vi "Configure Session.vi"(8 "error in":errorcluster, 11 "Plugin in":refnum<class "Sift Stream.lvclass">) -> (0 "error out":errorcluster, 3 "Plugin out":refnum<class "Sift Stream.lvclass">)   [LabVIEW 2024, in "Sift Stream.lvlib" / "Sift Stream.lvclass"]
uses:
  Sift Stream.lvclass
  C:/Program Files/National Instruments/LabVIEW 2024/vi.lib/FlexLogger/SDK/PluginSDK.lvlibp/PEFClasses/SDK/Plugin/Plugin.lvclass
  <vilib>/FlexLogger/SDK/PluginSDK.lvlibp/PEFClasses/SDK/Processing Element/Timing Parameters.ctl
  <vilib>/FlexLogger/SDK/PluginSDK.lvlibp/PEFClasses/SDK/Processing Element/Timing Method.ctl
  Sift Stream Parameters.ctl
  <vilib>/Sift/Sift/Sift API/Sift Client.lvclass
  Sift Stream.lvclass/Sift Stream.ctl
  <vilib>/FlexLogger/SDK/PluginSDK.lvlibp/PEFClasses/SDK/Plugin/ParameterAccess/Read String.vi
  <vilib>/FlexLogger/SDK/PluginSDK.lvlibp/PEFClasses/SDK/Plugin/ParameterAccess/Read DBL.vi
  <vilib>/FlexLogger/SDK/PluginSDK.lvlibp/PEFClasses/SDK/Plugin/ParameterAccess/Read N Channel.vi
  <vilib>/FlexLogger/SDK/PluginSDK.lvlibp/PEFClasses/SDK/Plugin/Plugin.lvclass
  <vilib>/FlexLogger/SDK/PluginSDK.lvlibp/PEFClasses/SDK/Processing Element/Processing Element.lvclass
  C:/Program Files/National Instruments/LabVIEW 2024/vi.lib/FlexLogger/SDK/PluginSDK.lvlibp/PEFClasses/SDK/Processing Element/Processing Element.lvclass
  C:/Users/Alex luCK/Documents/Projects/sift-labview/plugins/flexlogger/Sift Stream/source/Sift Stream/Sift Stream.lvclass
  <userlib>/_OpenG.lib/string/string.llb/openg_string.lvlib
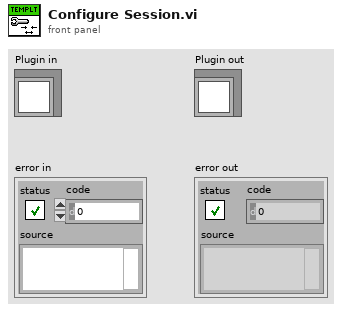
[diagram p1: front panel]
types:
  T1 = typedef "Sift Stream.lvlib/Sift Stream.lvclass/Sift Stream Parameters.ctl" = cluster{"API gRPC URL":string, "API REST URL":string, "API Key":string, "Asset Name":string, "Data Rate":dbl, "Stream Names":string[], "Sift Client":refnum<class "Sift Client.lvclass">, "Session Error":errorcluster}
  T2 = typedef "PluginSDK.lvlibp/Processing Element.lvclass/Timing Parameters.ctl" = cluster{"Timing Method":T3, "Timing Period (ms)":i32}
  T3 = typedef "PluginSDK.lvlibp/Processing Element.lvclass/Timing Method.ctl" = enum16{"Periodic", "Immediate", "On Data Ready", "Triggered"}
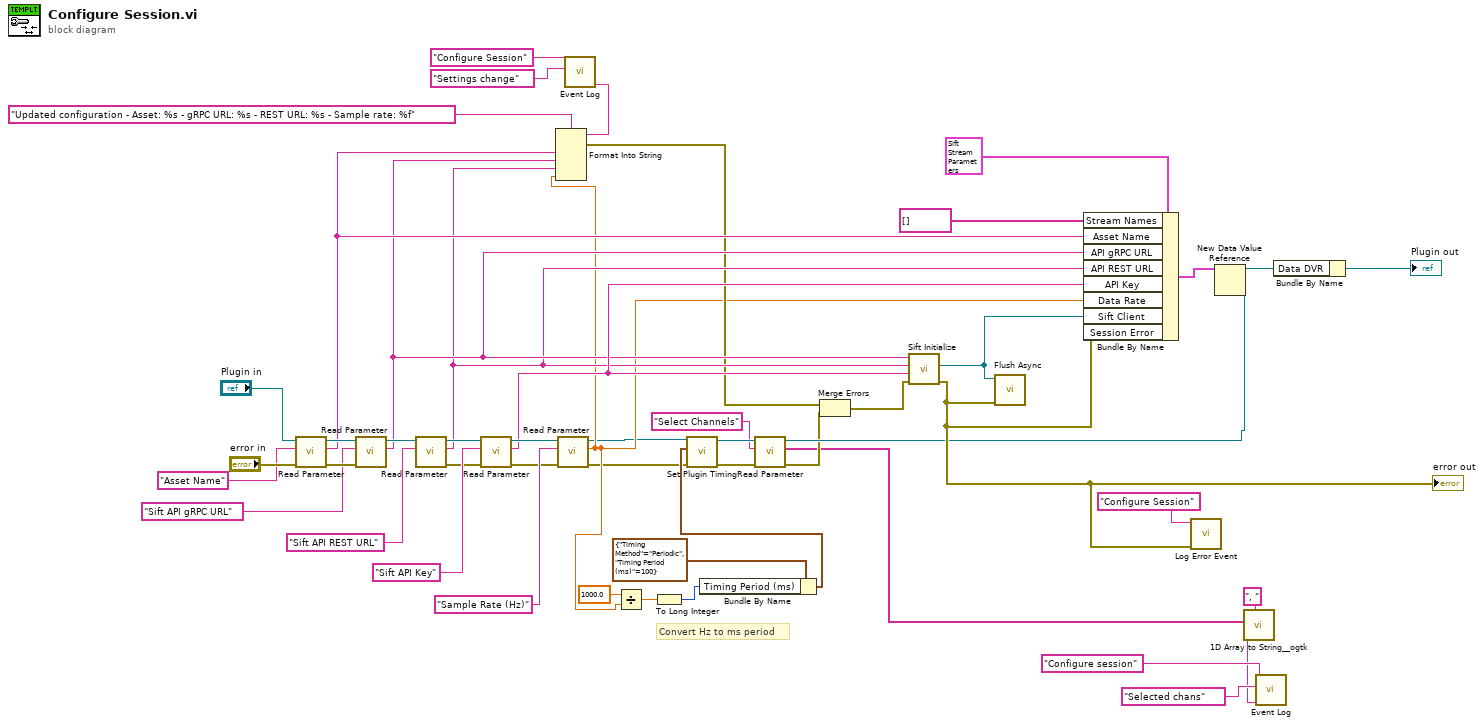
[diagram p0: block diagram]
diagram:
  # "Convert Hz to ms period"
  n1 = call-poly <vilib>:"Read Parameter.vi"("error in (no error)"="error in", "Name"="Asset Name", "Plugin in"="Plugin in") -> ("error out"=w45:errorcluster, "Value"=w27:string, "Plugin out"=w44:refnum<class "Sift Stream.lvclass">)  [unwired: 5 in, 1 out]
  n2 = call-poly <vilib>:"Read Parameter.vi"("error in (no error)"=w45, "Name"="Sift API gRPC URL", "Plugin in"=w44) -> ("Value"=w26:string, "Plugin out"=w43:refnum<class "Sift Stream.lvclass">)  [unwired: 5 in, 2 out]
  n3 = call-poly <vilib>:"Read Parameter.vi"("Name"="Sift API REST URL", "Plugin in"=w43) -> ("error out"=w37:errorcluster, "Value"=w25:string, "Plugin out"=w38:refnum<class "Sift Stream.lvclass">)  [unwired: 6 in, 1 out]
  n4 = call-poly <vilib>:"Read Parameter.vi"("error in (no error)"=w37, "Name"="Sift API Key", "Plugin in"=w38) -> ("error out"=w34:errorcluster, "Value"=w32:string, "Plugin out"=w35:refnum<class "Sift Stream.lvclass">)  [unwired: 5 in, 1 out]
  n5 = call-poly <vilib>:"Read Parameter.vi"("error in (no error)"=w34, "Name"="Sample Rate (Hz)", "Plugin in"=w35) -> ("error out"=w12:errorcluster, "Value"=w19:dbl, "Plugin out"=w11:refnum<class "Sift Stream.lvclass">)  [unwired: 5 in, 1 out]
  n6 = Format Into String(format string="Updated configuration - Asset: %s - gRPC URL: %s - REST URL: %s - Sample rate: %f", w27, w26, w25, w19) -> (resulting string=w21:string, error out=w23:errorcluster)  [unwired: 2 in]
  n7 = call "Event Log.vi"("Message"=w21, "Event Type"="Settings change", "Location"="Configure Session") -> ()  [unwired: 9 in]
  n8 = Divide(x=1000.0, y=w19) -> (x/y=w17:dbl)
  n9 = To Long Integer(number=w17) -> (32bit integer=w15:i32)
  n10 = Bundle By Name(cluster=T2 {"Timing Method"=enum."Periodic", "Timing Period (ms)"=100} ("Timing Parameters"), "Timing Period (ms)"=w15) -> (w14:T2)
  n11 = call <vilib>:"Set Plugin Timing.vi"("error in (no error)"=w12, "Timing Parameters"=w14, "Plugin in"=w11) -> ("error out"=w10:errorcluster, "Plugin out"=w9:refnum<class "Sift Stream.lvclass">)  [unwired: 7 in]
  n12 = call-poly <vilib>:"Read Parameter.vi"("error in (no error)"=w10, "Name (Unique Channel Identifier)"="Select Channels", "Plugin in"=w9) -> ("error out"=w7:errorcluster, "Channels"=w2:string[], "Plugin out"=w8:refnum<class "Sift Stream.lvclass">)  [unwired: 5 in, 1 out]
  n13 = Merge Errors(w23, w7) -> (w22:errorcluster)
  n14 = call "Sift Initialize.vi"("error in"=w22, "API Key"=w32, "API REST URL"=w25, "API gRPC URL"=w26) -> ("error out"=w13:errorcluster, "Sift Client out"=w30:refnum<class "Sift Client.lvclass">)  [unwired: 4 in]
  "error out" <- w13
  n15 = call "Flush Async.vi"("error in (no error)"=w13, "Sift Client In"=w30) -> ()  [unwired: 10 in]
  n16 = Bundle By Name(cluster=T1 {"API gRPC URL"="", "API REST URL"="", "API Key"="", "Asset Name"="", "Data Rate"=0.0, "Stream Names"=[], "Sift Client"=refnum, "Session Error"={"status"=FALSE, "code"=0, "source"=""}} ("StreamWriter Parameters"), "Stream Names"=string[] [], "Asset Name"=w27, "API gRPC URL"=w26, "API REST URL"=w25, "API Key"=w32, "Data Rate"=w19, "Sift Client"=w30, "Session Error"=w13) -> (w50:T1)
  n17 = call "Log Error Event.vi"("error in (no error)"=w13, "Location"="Configure Session") -> ()  [unwired: 10 in]
  n18 = New Data Value Reference(data value=w50) -> (data value reference=w31:refnum<data-value>)  [unwired: 1 in, 1 out]
  n19 = call <userlib>:"1D Array to String__ogtk.vi"("delimiter (Tab)"=", ", "Array of Strings"=w2) -> ("delimited string"=w3:string)  [unwired: 9 in]
  n20 = call "Event Log.vi"("Message"=w3, "Event Type"="Selected chans", "Location"="Configure session") -> ()  [unwired: 9 in]
  n21 = Bundle By Name(cluster=w8, "Data DVR"=w31) -> (→"Plugin out":refnum<class "Sift Stream.lvclass">)
